vi "Append (double scaler).vi"(6 "Reset":bool, 8 "error in (no error)":errorcluster, 9 "Y":dbl, 10 "X":dbl, 11 "XY-data (A)":cluster{"X-array":dbl[], "Y-array":dbl[]}) -> (0 "error out":errorcluster, 3 "XY-data out":cluster{"X-array":dbl[], "Y-array":dbl[]} {"Y-array" format="%.2p"; "X-array" format="%.2p"})   [LabVIEW 2019, in "xy_utilities.lvlib"]
doc: "Append <B>XY-Data B</B> to the end of <B>XY-Data A</B> (similar to Append Waveforms.vi).\n\nWire data to the data input to determine the polymorphic instance to use or manually select the instance."
uses:
  xy_utilities.lvlib
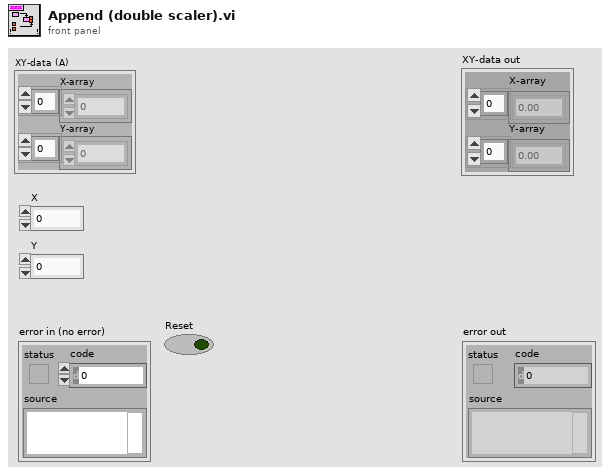
[diagram p1: front panel]
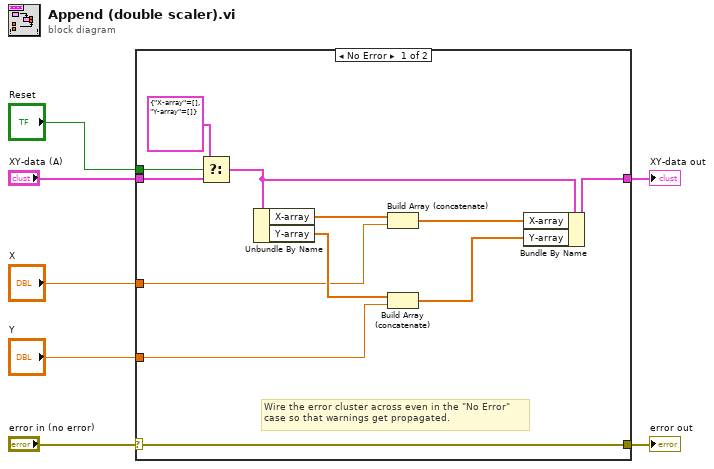
[diagram p0: block diagram]
diagram:
  n1 = case shown="No Error" "error in (no error)" {
    selector: "error in (no error)" -> [w19 w21]
    tunnel: [w19 w21] -> w6
    tunnel: "XY-data (A)" -> [w10 w20]
    tunnel: [w18 w20] -> w4
    tunnel: "X" -> [w13 _]
    tunnel: "Y" -> [w12 _]
    tunnel: "Reset" -> [w11 _]
    frame No Error {
      # "Wire the error cluster across even in the \"No Error\"\ncase so that warnings get propagated."
      n2 = Select(t=cluster{"X-array":dbl[], "Y-array":dbl[]} {"X-array"=[], "Y-array"=[]} ("XY-data (A)"), s=w11, f=w10) -> (s? t:f=w9:cluster{"X-array":dbl[], "Y-array":dbl[]})
      n3 = Unbundle By Name(w9) -> ("X-array"=w17:dbl[], "Y-array"=w15:dbl[])
      n4 = Build Array (concatenate)(w17, w13) -> (w16:dbl[])
      n5 = Build Array (concatenate)(w15, w12) -> (w14:dbl[])
      n6 = Bundle By Name(cluster=w9, "X-array"=w16, "Y-array"=w14) -> (w18:cluster{"X-array":dbl[], "Y-array":dbl[]})
    }
    frame Error {
    }
  }
  "error out" <- w6
  "XY-data out" <- w4
